vi "ClosePhotoDetector.vi"(8 "error in (no error)":errorcluster, 11 "instrument handle":refnum<visa-resource-name>) -> (3 "error out":errorcluster)   [LabVIEW 2018]
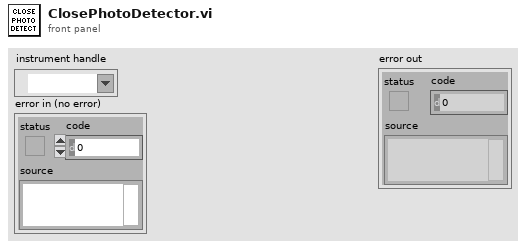
[diagram p1: front panel]
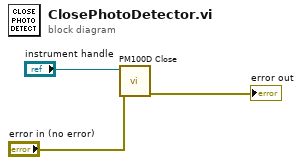
[diagram p0: block diagram]
diagram:
  n1 = call "PM100D Close.vi"("error in (no error)"="error in (no error)", "instrument handle"="instrument handle") -> ("error out"=→"error out":errorcluster)  [unwired: 9 in]
